vi "Kinematic tester.vi"() -> ()   [LabVIEW 2013]
uses:
  <vilib>/Analysis/Matrix/Datatypes/RealMatrix.ctl
  ROS/Code/SubVIs/BaxterSide.ctl
  ROS/Code/Console/Servers/ServerSubs/(nist) Arm Globals.vi
  Fwd Kenimatics - array.vi
  <vilib>/Analysis/Matrix/NI_Matrix.lvlib
panel:
  in  "R:Joints 2":dbl[](array[numeric])=[-40.0, -65.0, 0.0, 100.0, 0.0, 75.0, 0.0]
  out "Matrix":T1=[[-0.08414709700680022, 0.9964531157860806, 0.0006738735338379292, 52.018089073754005], [0.9964530496622023, 0.08414653345687258, 0.0008250612629564553, -888.1364716299727], [0.0007654307443265374, 0.0007409098480100078, -0.9999994325840253, 173.90623351008412], [0.0, 0.0, 0.0, 1.0]] format="%.3f"
  out "Found":bool=TRUE
  out "R:Joints":dbl[](array[numeric])=[-40.14404292287874, -64.95117180078246, -0.08789062489957031, 90.04394520960979, 0.08789062489957031, 64.95117180078246, -0.08789062489957031]
  out "J":dbl[](array[numeric])=[-40.0, -64.9609375, -0.29296875, 90.05859375, 0.18365400555870967, 64.94666842723873, -0.1702843404592511] format="%.3f"
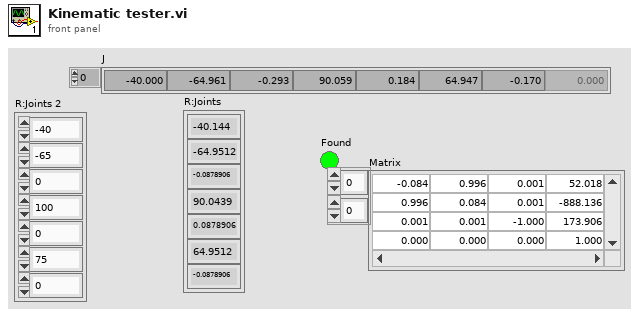
[diagram p1: front panel]
types:
  T1 = typedef "NI_Matrix.lvlib/RealMatrix.ctl" = dbl[][]
  T2 = typedef "BaxterSide.ctl" = enum16{"left", "right"}
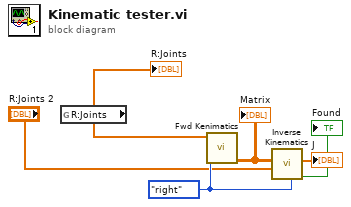
[diagram p0: block diagram]
diagram:
  w2 = BaxterSide."right" ("Side")
  n1 = global read "(nist) Arm Globals.vi" "R:Joints"() -> (w5:dbl[])
  "R:Joints" <- w5
  n2 = call-poly "Fwd Kenimatics.vi"("Side"=w2, "Joints"=w5) -> ("Matrix"=w6:T1)  [unwired: 8 in, 1 out]
  "Matrix" <- w6
  n3 = call "Inverse Kinematics.vi"("Side"=w2, "Start"="R:Joints 2", "Goal-matrix"=w6) -> ("Found"=→"Found":bool, "J"=→"J":dbl[])  [unwired: 5 in, 2 out]
